vi "Default Settings.vi"(8 "error in (no error)":errorcluster, 11 "C4 Dispense in 2":refnum<class "6 Inch Iterative Dispense.lvclass">) -> (0 "error out":errorcluster, 3 "C4 Dispense out 2":refnum<class "6 Inch Iterative Dispense.lvclass">)   [LabVIEW 2019, in "6 Inch Iterative Dispense.lvclass"]
uses:
  6 Inch Iterative Dispense.lvclass
  C:/Users/HEP/Documents/Aerotech gantry/UCSB-Gantry-master-main/V5/Classes/Routine/Dispense/Iterative Dispense/Iterative Dispense.lvclass
  C:/Users/HEP/Documents/Aerotech gantry/UCSB-Gantry-master-main/V5/Classes/Routine/Dispense/Dispense.lvclass
  Iterative Dispense.lvclass/Iterative Dispense.ctl
  Read Speed.vi
  Read Number of Lines.vi
  Read Distance From Edges.vi
  Iterative Dispense.lvclass
  Dispense.lvclass
panel:
  # "This Routine does not Accept Settings"
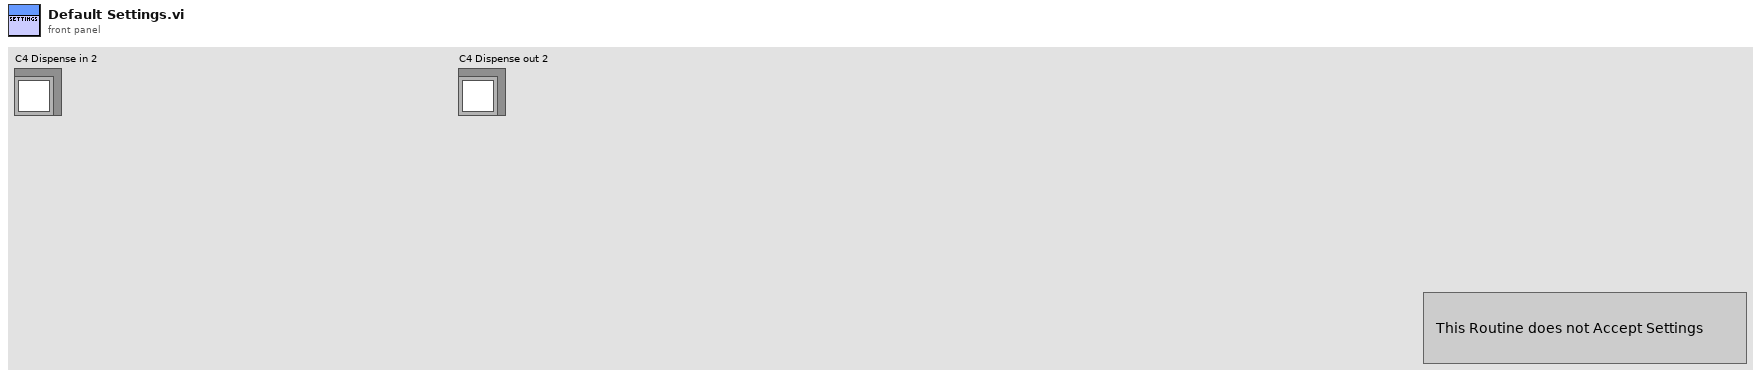
[diagram p1: front panel]
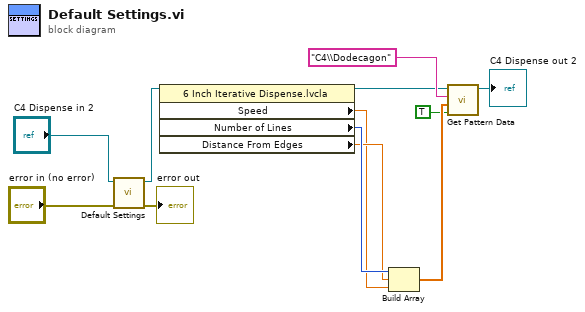
[diagram p0: block diagram]
diagram:
  n1 = call-parent "Default Settings.vi"("error in (no error)"="error in (no error)", "C4 Dispense in 2"="C4 Dispense in 2") -> ("error out"=→"error out":errorcluster, "C4 Dispense out 2"=w9:refnum<class "6 Inch Iterative Dispense.lvclass">)  [unwired: 8 in]
  n2 = property class="6 Inch Iterative Dispense.lvcla"(reference=w9) -> (reference out=w7:refnum<class "6 Inch Iterative Dispense.lvclass">, "Speed"=w3:dbl, "Number of Lines"=w5:i32, "Distance From Edges"=w4:dbl)  [unwired: 1 in, 1 out]
  n3 = Build Array(w5, w4, w3) -> (w2:dbl[])
  n4 = call "Get Pattern Data.vi"("Iterative?"=TRUE, "File Name"=w2, "Folder Name"="C4\\Dodecagon", "Dispense.lvclass"=w7) -> ("Dispense Out"=→"C4 Dispense out 2":refnum<class "6 Inch Iterative Dispense.lvclass">)  [unwired: 7 in]
